vi "Check_and_Modify_Statuses_101_Case-1.vi"(4 "[IN] Number of Co\nnnected Points":i32, 6 "[IN] Index of Po\nint After \"101\"":i32, 7 "[IN] Index of Pro\nblem \"101\" Point":i32, 8 "[IN] Current Index":i32, 9 "[IN] Current Status":i16) -> (3 "[OUT] Status":i16)   [LabVIEW 2013]
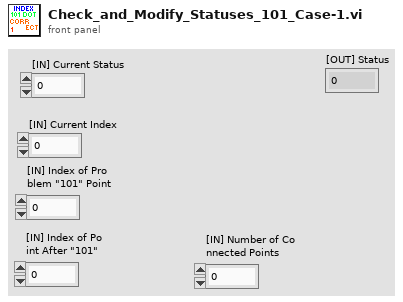
[diagram p1: front panel]
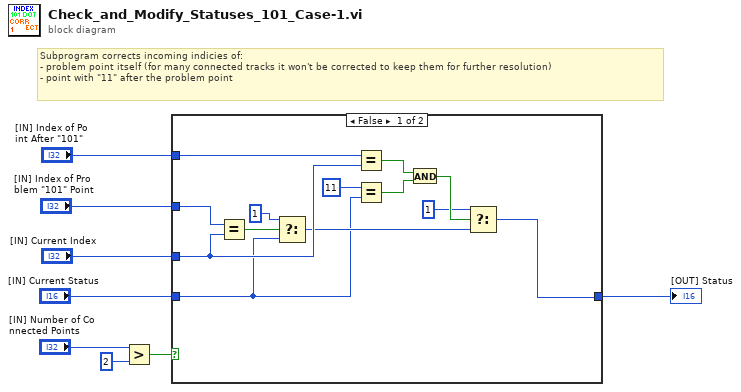
[diagram p0: block diagram]
diagram:
  # "Subprogram corrects incoming indicies of:\n- problem point itself (for many connected tracks it won't be corrected to keep them for further resolution)\n- point with \"11\" after the problem point"
  n1 = Greater?(x="[IN] Number of Co\nnnected Points", y=2) -> (0:w6:bool)
  n2 = case shown="False" w6 {
    tunnel: "[IN] Index of Pro\nblem \"101\" Point" -> [w21 _]
    tunnel: "[IN] Current Index" -> [w17 _]
    tunnel: "[IN] Current Status" -> [w11 w22]
    tunnel: "[IN] Index of Po\nint After \"101\"" -> [w18 _]
    tunnel: [w9 w22] -> w1
    frame False {
      n3 = Equal?(x=w21, y=w17) -> (x = y?=w20:bool)
      n4 = Select(t=i16 1, s=w20, f=w11) -> (s? t:f=w13:i16)
      n5 = Equal?(x=w18, y=w17) -> (x = y?=w10:bool)
      n6 = Equal?(x=i16 11, y=w11) -> (x = y?=w15:bool)
      n7 = And(x=w10, y=w15) -> (x .and. y?=w14:bool)
      n8 = Select(t=i16 1, s=w14, f=w13) -> (s? t:f=w9:i16)
    }
    frame True {
    }
  }
  "[OUT] Status" <- w1
